vi "Read Count.vi"(8 "error in (no error)":errorcluster, 11 "Repeat Until Count in":refnum<class "Repeat Until Count.lvclass">) -> (0 "error out":errorcluster, 2 "Count":i32, 3 "Repeat Until Count out":refnum<class "Repeat Until Count.lvclass">)   [LabVIEW 2021, in "BT.lvlib" / "Repeat Until Count.lvclass"]
uses:
  Repeat Until Count.lvclass
  Repeat Until Count.lvclass/Repeat Until Count.ctl
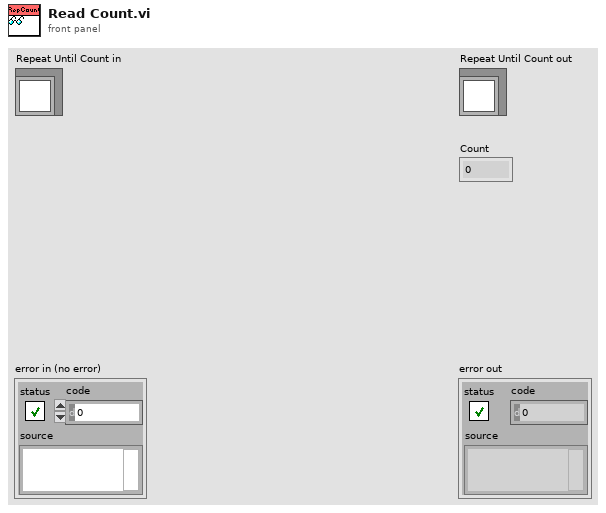
[diagram p1: front panel]
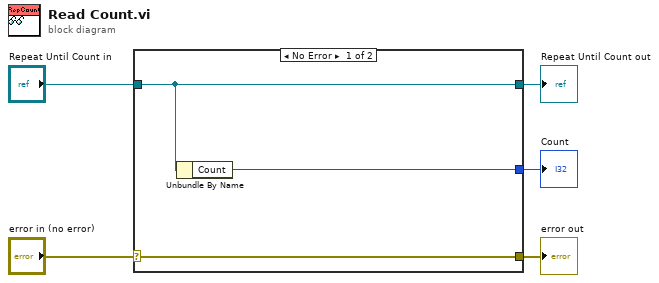
[diagram p0: block diagram]
diagram:
  n1 = case shown="No Error" "error in (no error)" {
    selector: "error in (no error)" -> [w8 w9]
    tunnel: [w8 w9] -> w4
    tunnel: [w7 w10] -> w2
    tunnel: "Repeat Until Count in" -> [w7 w10]
    tunnel: [w6 _] -> w1
    frame No Error {
      n2 = Unbundle By Name(w7) -> ("Count"=w6:i32)
    }
    frame Error {
    }
  }
  "error out" <- w4
  "Repeat Until Count out" <- w2
  "Count" <- w1
